vi "updated_hai-3.vi"() -> ()   [LabVIEW 2023]
uses:
  <vilib>/Utility/NIReport.llb/Report Type.ctl
  <vilib>/Utility/NIReport.llb/Append Text Table to Report (wrap).vi
  <vilib>/Utility/NIReport.llb/NI_report.lvclass
  <vilib>/Utility/NIReport.llb/NI_ReportGenerationCore.lvlib
  <vilib>/Utility/NIReport.llb/Excel/NI_Excel.lvclass
panel:
  out "Remaining_hours(hrs)":dbl
  out "Current flow out rate":dbl
  out "Current flow in rate":dbl
  out "Current water level  in litres:":dbl
  in  "Flow out rate(litres/sec)":dbl(slide) scale=0.0..25.0
  in  "Flow in rate(liters/sec)":dbl(slide) step=1.0 scale=0.0..10.0
  out "Water level is low":bool
  out "Water level is high":bool
  out "Tank":dbl(slide) scale=0.0..10000.0
  in  "stop":bool
  in  "report file path":path
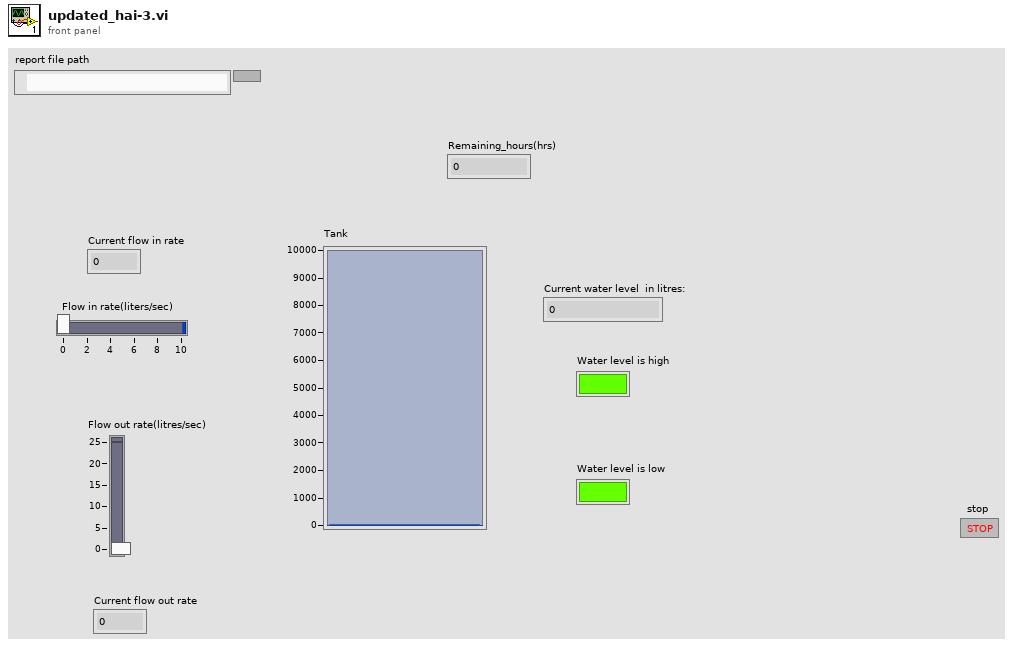
[diagram p1: front panel]
types:
  T1 = typedef "NI_ReportGenerationCore.lvlib/Report Type.ctl" = enum16{"HTML", "Word", "Excel"}
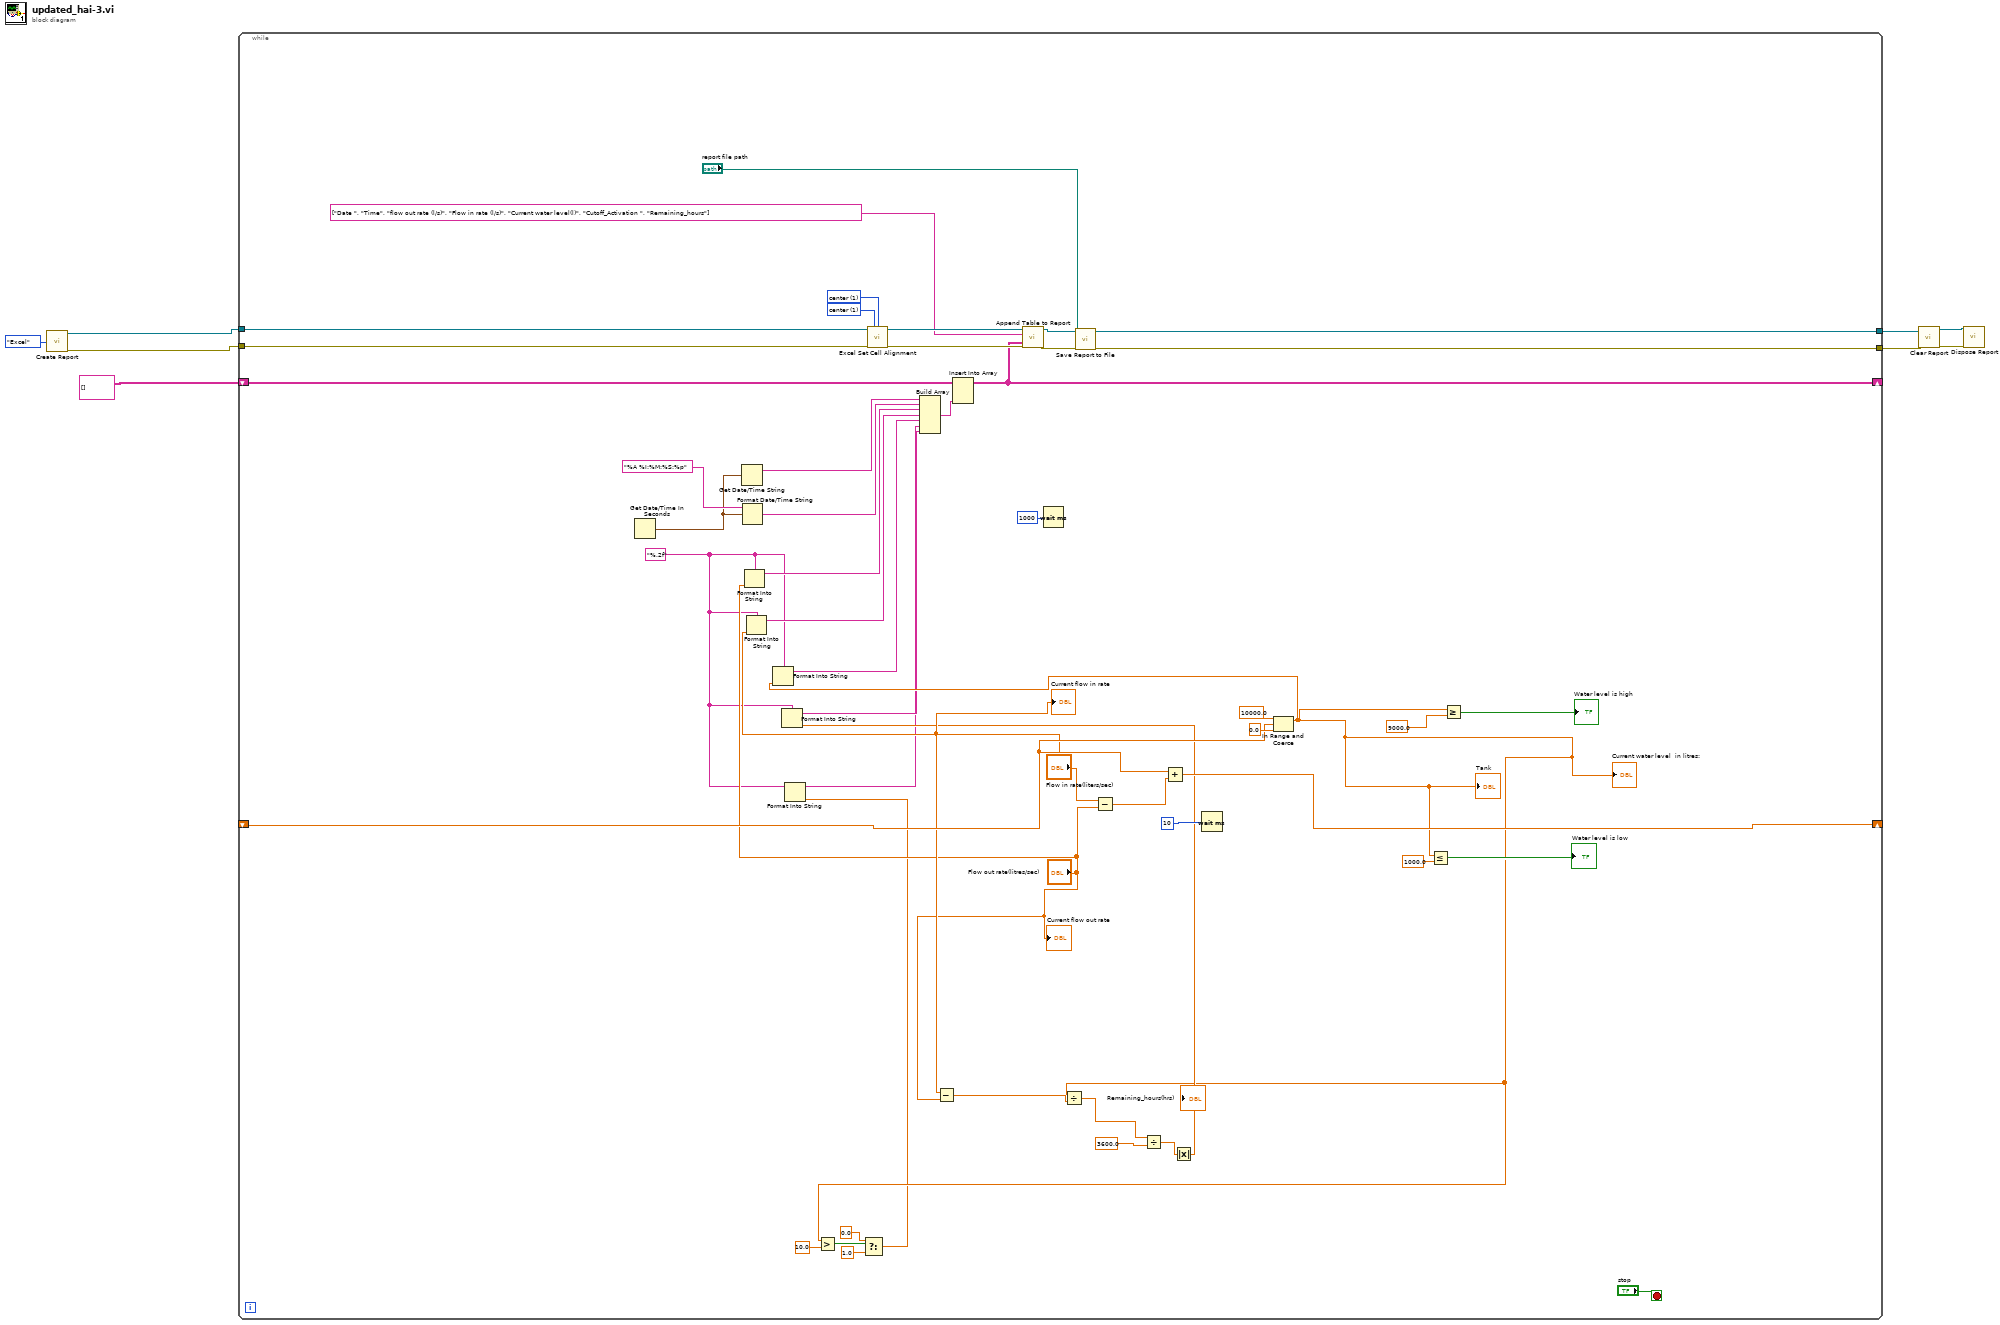
[diagram p0: block diagram]
diagram:
  n1 = call <vilib>:"Create Report.vi"("report type"=Report_Type."Excel") -> ("report out"=w7:refnum<class "NI_report.lvclass">, "error out"=w6:errorcluster)  [unwired: 13 in]
  n2 = while {
    tunnel: w7 -> [w58]
    tunnel: w6 -> [w57]
    tunnel: [w50] -> w5
    tunnel: [w49] -> w4
    shift-right: [w40] -> _
    shift-left: string[][] [] -> [w41]
    shift-right: [w27] -> _
    shift-left: _ -> [w26]
    stop <- "stop" stop-if-true
    w15 = "%.2f" ("format string")
    w55 = 1 items=["left", "center", "right"] ("horizontal alignment (left)")
    w56 = 1 items=["top", "center", "bottom"] ("vertical alignment (top)")
    n3 = Get Date/Time In Seconds() -> (seconds since 1Jan1904=w47:timestamp)
    n4 = Get Date/Time String(seconds (now)=w47) -> (date string=w46:string)  [unwired: 2 in, 1 out]
    n5 = Format Date/Time String(time format string (%c)="%A %I:%M:%S:%p", seconds (now)=w47) -> (date/time string=w45:string)  [unwired: 1 in]
    n6 = Format Into String(format string=w15, "Flow out rate(litres/sec)") -> (resulting string=w44:string)  [unwired: 2 in, 1 out]
    n7 = Format Into String(format string=w15, "Flow in rate(liters/sec)") -> (resulting string=w43:string)  [unwired: 2 in, 1 out]
    n8 = call <vilib>:"Excel Set Cell Alignment.vi"("report in"=w58, "vertical alignment (top)"=w56, "horizontal alignment (left)"=w55, "error in (no error)"=w57) -> ("report out"=w54:refnum<class "NI_report.lvclass">, "error out"=w53:errorcluster)  [unwired: 10 in]
    n9 = Subtract(x="Flow in rate(liters/sec)", y="Flow out rate(litres/sec)") -> (x-y=w22:dbl)
    n10 = Wait (ms)(milliseconds to wait=u32 1000) -> ()  [unwired: 1 out]
    n11 = Subtract(x="Flow in rate(liters/sec)", y="Flow out rate(litres/sec)") -> (x-y=w35:dbl)
    n12 = Add(x=w26, y=w35) -> (x+y=w27:dbl)
    n13 = Wait (ms)(milliseconds to wait=u32 10) -> ()  [unwired: 1 out]
    n14 = In Range and Coerce(upper limit=10000.0, x=w26, lower limit=0.0) -> (coerced(x)=w19:dbl)  [unwired: 1 out]
    "Tank" <- w19
    "Current water level  in litres:" <- w19
    n15 = Format Into String(format string=w15, w19) -> (resulting string=w25:string)  [unwired: 2 in, 1 out]
    n16 = Greater?(x=w19, y=10.0) -> (0:w18:bool)
    n17 = Select(t=0.0, s=w18, f=1.0) -> (s? t:f=w14:dbl)
    n18 = Format Into String(format string=w15, w14) -> (resulting string=w12:string)  [unwired: 2 in, 1 out]
    n19 = Divide(x=w19, y=w22) -> (x/y=w11:dbl)
    n20 = Divide(x=w11, y=3600.0) -> (x/y=w9:dbl)
    n21 = Absolute Value(x=w9) -> (abs(x)=w21:dbl)
    "Remaining_hours(hrs)" <- w21
    n22 = Format Into String(format string=w15, w21) -> (resulting string=w13:string)  [unwired: 2 in, 1 out]
    n23 = Build Array(w46, w45, w44, w43, w25, w12, w13) -> (w42:string[])
    n24 = Insert Into Array(array=w41, new element=w42) -> (w40:string[][])  [unwired: 2 in]
    n25 = call-poly <vilib>:"Append Table to Report.vi"("report in"=w54, "column headers"=string[] ["Date ", "Time", "flow out rate (l/s)", "Flow in rate (l/s)", "Current water level(l)", "Cutoff_Activation ", "Remaining_hours"] ("row headers"), "text data"=w40, "error in (no error)"=w53) -> ("report out"=w52:refnum<class "NI_report.lvclass">, "error out"=w51:errorcluster)  [unwired: 8 in, 2 out]
    n26 = call-dynamic "Save Report to File.vi"("report in"=w52, "report file path"="report file path", "error in (no error)"=w51) -> ("report out"=w50:refnum<class "NI_report.lvclass">, "error out"=w49:errorcluster)  [unwired: 11 in]
    n27 = Less Or Equal?(x=w19, y=1000.0) -> (x <= y?=→"Water level is low":bool)
    n28 = Greater Or Equal?(x=w19, y=9000.0) -> (x >= y?=→"Water level is high":bool)
    "Current flow in rate" <- "Flow in rate(liters/sec)"
    "Current flow out rate" <- "Flow out rate(litres/sec)"
  }
  n29 = call-dynamic "Clear Report.vi"("report in"=w5, "error in (no error)"=w4) -> ("report out"=w3:refnum<class "NI_report.lvclass">, "error out"=w2:errorcluster)  [unwired: 12 in]
  n30 = call-dynamic "Dispose Report.vi"("report in"=w3, "error in (no error)"=w2) -> ()  [unwired: 13 in, 1 out]
